vi "testPreserveRawXml.vi"(8 "error in (no error)":errorcluster, 11 "TestCase in":refnum<class "EasyXMLTest.lvclass">) -> (0 "error out":errorcluster, 3 "TestCase out":refnum<class "EasyXMLTest.lvclass">)   [LabVIEW 2011, in "EasyXMLTest.lvclass"]
doc: "Verify that error in is not overwritten"
uses:
  EasyXMLTest.lvclass
  <userlib>/_OpenG.lib/string/string.llb/Convert EOLs (String)__ogtk.vi
panel:
  out "generated \"sub\" substring":string
  out "\"sub\" substring":string="hello"
  out "XML String":string
  out "Generated XML String":string
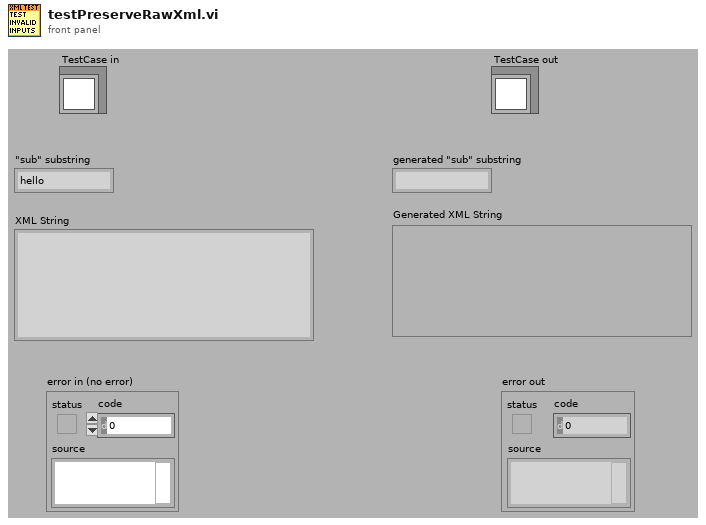
[diagram p1: front panel]
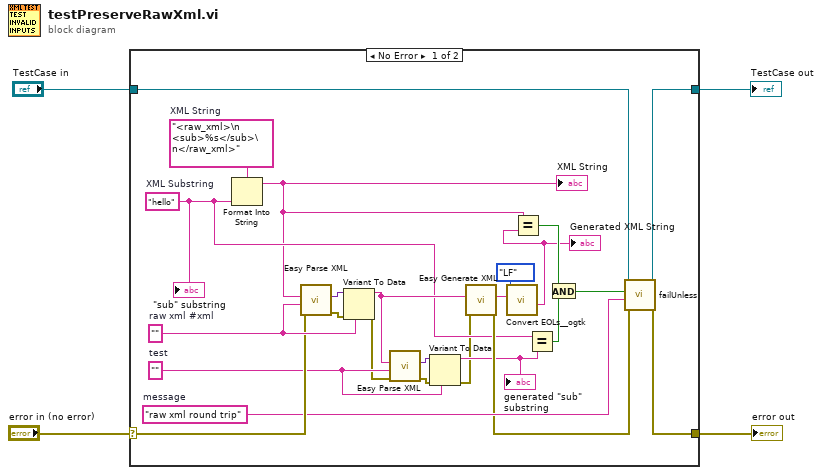
[diagram p0: block diagram]
diagram:
  n1 = case shown="No Error" "error in (no error)" {
    selector: "error in (no error)" -> [w26 w31]
    tunnel: [w17 w31] -> w2
    tunnel: [w19 w30] -> w1
    tunnel: "TestCase in" -> [w20 w30]
    frame No Error {
      w13 = "hello"  # XML Substring
      w21 = ""  # test
      w27 = ""  # raw xml #xml
      w15 = "<raw_xml>\n  <sub>%s</sub>\n</raw_xml>"  # XML String
      w25 = "raw xml round trip"  # message
      n2 = Format Into String(format string=w15, w13) -> (resulting string=w8:string)  [unwired: 2 in, 1 out]
      "XML String" <- w8
      n3 = call "Easy Parse XML.vi"("error in (no error)"=w26, "LabVIEW Data (Type)"=w27, "XML String"=w8) -> ("error out"=w28:errorcluster, "LabVIEW Data"=w29:variant)  [unwired: 7 in]
      n4 = Variant To Data(error in=w28, type=w27, Variant=w29) -> (data=w24:string, error out=w16:errorcluster)
      n5 = call "Easy Parse XML.vi"("error in (no error)"=w16, "LabVIEW Data (Type)"=w21, "XML String"=w24) -> ("error out"=w23:errorcluster, "LabVIEW Data"=w22:variant)  [unwired: 7 in]
      n6 = Variant To Data(error in=w23, type=w21, Variant=w22) -> (data=w14:string, error out=w9:errorcluster)
      "generated \"sub\" substring" <- w14
      n7 = call "Easy Generate XML.vi"("error in (no error)"=w9, "LabVIEW Data"=w24) -> ("error out"=w18:errorcluster, "XML String"=w7:string)  [unwired: 8 in]
      n8 = call-poly <userlib>:"Convert EOLs__ogtk.vi"("Convert to:"=enum16{"CR", "LF", "CRLF"}."LF", "String in"=w7) -> ("String out"=w6:string)  [unwired: 9 in]
      "Generated XML String" <- w6
      n9 = Equal?(x=w8, y=w6) -> (x = y?=w11:bool)
      n10 = Equal?(x=w13, y=w14) -> (x = y?=w12:bool)
      n11 = And(x=w11, y=w12) -> (x .and. y?=w10:bool)
      n12 = call-dynamic "failUnless.vi"("error in (no error)"=w18, "message (\"\")"=w25, "pass"=w10, "TestCase in"=w20) -> ("error out"=w17:errorcluster, "TestCase out"=w19:refnum<class "EasyXMLTest.lvclass">)  [unwired: 6 in]
      "\"sub\" substring" <- w13
    }
    frame Error {
    }
  }
  "error out" <- w2
  "TestCase out" <- w1
